vi "Read Local Personality File.vi"(8 "error in (no error)":errorcluster, 11 "File Path":path) -> (0 "error out":errorcluster, 3 "Personality text":string, 5 "path":path)   [LabVIEW 2018, in "Personalities Tool.lvlib"]
doc: "This VI opens a file and retuns its contents."
uses:
  Personalities Tool.lvlib
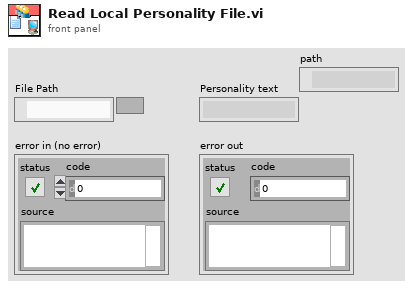
[diagram p1: front panel]
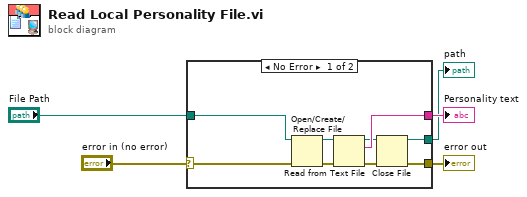
[diagram p0: block diagram]
diagram:
  n1 = case shown="No Error" "error in (no error)" {
    selector: "error in (no error)" -> [w12 w16]
    tunnel: "File Path" -> [w7 w15]
    tunnel: [w14 _] -> w4
    tunnel: [w13 w16] -> w3
    tunnel: [w6 w15] -> w1
    frame No Error {
      n2 = Open/Create/Replace File(file path (use dialog)=w7, error in=w12) -> (refnum out=w8:refnum<file>, error out=w9:errorcluster)  [unwired: 4 in, 1 out]
      n3 = Read from Text File(file (use dialog)=w8, error in=w9) -> (refnum out=w10:refnum<file>, text=w14:string, error out=w11:errorcluster)  [unwired: 2 in, 1 out]
      n4 = Close File(refnum=w10, error in=w11) -> (path=w6:path, error out=w13:errorcluster)
    }
    frame Error {
    }
  }
  "Personality text" <- w4
  "error out" <- w3
  "path" <- w1
